vi "Get Commd.vi"(8 "error in (no error)":errorcluster, 11 "Channel in":refnum<class "Channel.lvclass">) -> (0 "error out":errorcluster, 3 "Channel out":refnum<class "Channel.lvclass">)   [LabVIEW 2018, in "Channel.lvclass"]
doc: "Remove from the qeue the last command sent by the control interface"
uses:
  Channel.lvclass
  Channel.lvclass/Channel.ctl
  RxTx/RxTx.lvclass
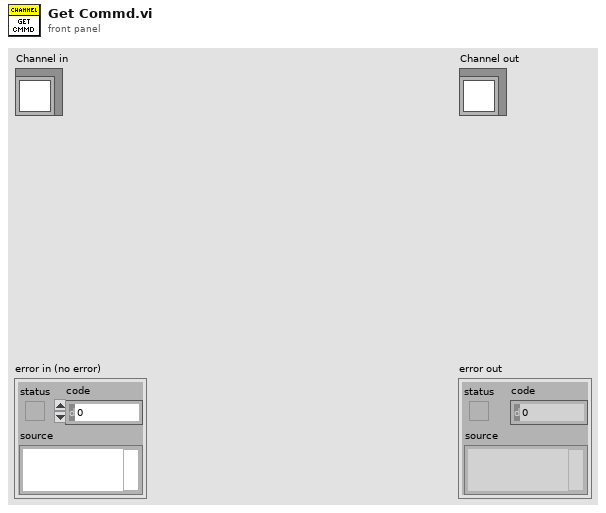
[diagram p1: front panel]
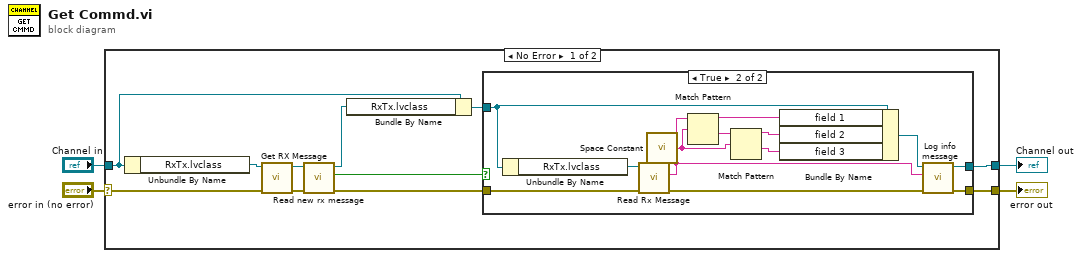
[diagram p0: block diagram]
diagram:
  n1 = case shown="No Error" "error in (no error)" {
    selector: "error in (no error)" -> [w14 w32]
    tunnel: [w10 w32] -> w3
    tunnel: [w11 w31] -> w1
    tunnel: "Channel in" -> [w13 w31]
    frame No Error {
      n2 = Unbundle By Name(w13) -> ("RxTx.lvclass"=w15:refnum<class "RxTx.lvclass">)
      n3 = call "Get RX Message.vi"("error in (no error)"=w14, "RxTx in"=w15) -> ("error out"=w7:errorcluster, "RxTx out"=w9:refnum<class "RxTx.lvclass">)  [unwired: 8 in]
      n4 = call-dynamic "Read new rx message.vi"("error in (no error)"=w7, "RxTx in"=w9) -> ("error out"=w6:errorcluster, "new rx message"=w5:bool, "RxTx out"=w8:refnum<class "RxTx.lvclass">)  [unwired: 7 in]
      n5 = Bundle By Name(cluster=w13, "RxTx.lvclass"=w8) -> (w12:refnum<class "Channel.lvclass">)
      n6 = case shown="True" w5 {
        tunnel: w12 -> [w17 w30]
        tunnel: [w17 w18] -> w11
        tunnel: [w16 w20] -> w10
        tunnel: w6 -> [w16 w23]
        frame False {
        }
        frame True {
          n7 = Unbundle By Name(w30) -> ("RxTx.lvclass"=w24:refnum<class "RxTx.lvclass">)
          n8 = call "Read Rx Message.vi"("error in (no error)"=w23, "RxTx in"=w24) -> ("error out"=w21:errorcluster, "Rx Message"=w22:string)  [unwired: 7 in, 1 out]
          n9 = call <vilib>:"Space Constant.vi"() -> ("String"=w28:string)
          n10 = Match Pattern(string=w22, regular expression=w28) -> (before substring=w27:string, after substring=w29:string)  [unwired: 1 in, 2 out]
          n11 = Match Pattern(string=w29, regular expression=w28) -> (before substring=w26:string, after substring=w25:string)  [unwired: 1 in, 2 out]
          n12 = Bundle By Name(cluster=w30, "field 1"=w27, "field 2"=w26, "field 3"=w25) -> (w19:refnum<class "Channel.lvclass">)
          n13 = call "Log info message.vi"("error in (no error)"=w21, "String"=w22, "Channel in"=w19) -> ("error out"=w20:errorcluster, "Channel out"=w18:refnum<class "Channel.lvclass">)  [unwired: 7 in]
        }
      }
    }
    frame Error {
    }
  }
  "error out" <- w3
  "Channel out" <- w1
